vi "Geraete Type ermitteln.vi"(8 "error in (no error)":errorcluster caption="Fehler (Eingang, kein Fehler)", 10 "Istwerte":u16[](array[numeric]), 11 "Steuerung PNS Eingang":refnum<class "Steuerung PNS.lvclass">) -> (0 "error out":errorcluster caption="Fehler (Ausgang)", 2 "Gerätetype":string, 3 "Steuerung PNS Ausgang":refnum<class "Steuerung PNS.lvclass">)   [LabVIEW 2020, in "Steuerung PNS.lvclass"]
uses:
  Steuerung PNS.lvclass
  Steuerung PNS.lvclass/Steuerung PNS.ctl
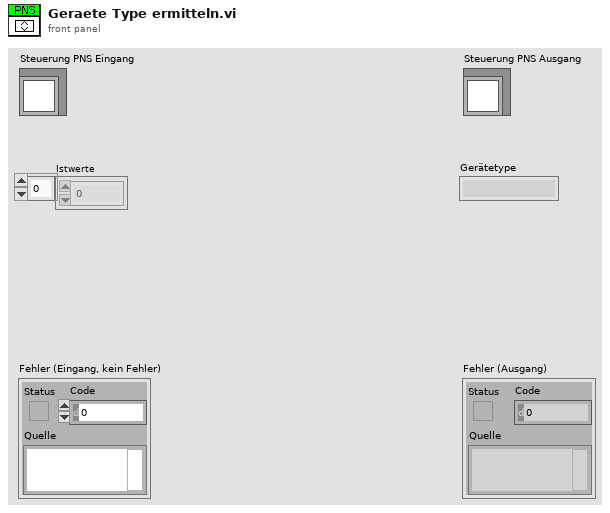
[diagram p1: front panel]
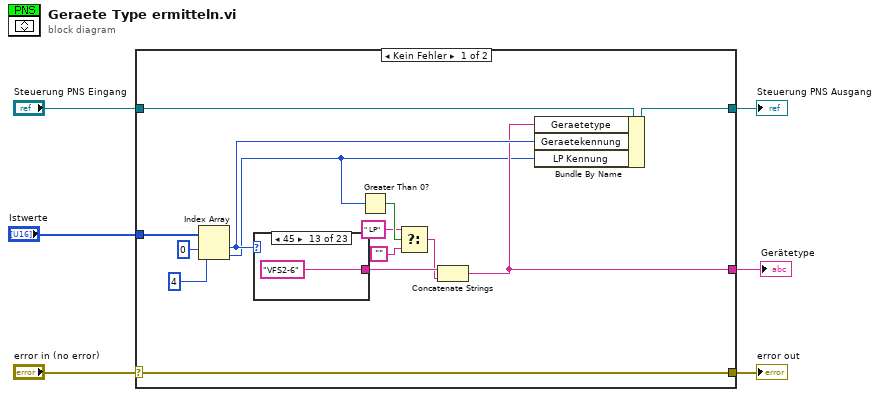
[diagram p0: block diagram]
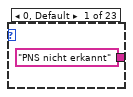
[diagram p2: hidden frame]
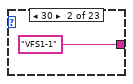
[diagram p3: hidden frame]
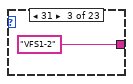
[diagram p4: hidden frame]
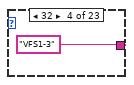
[diagram p5: hidden frame]
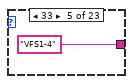
[diagram p6: hidden frame]
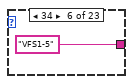
[diagram p7: hidden frame]
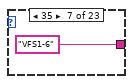
[diagram p8: hidden frame]
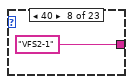
[diagram p9: hidden frame]
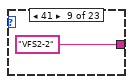
[diagram p10: hidden frame]
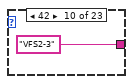
[diagram p11: hidden frame]
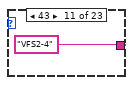
[diagram p12: hidden frame]
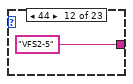
[diagram p13: hidden frame]
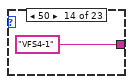
[diagram p14: hidden frame]
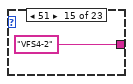
[diagram p15: hidden frame]
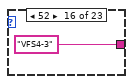
[diagram p16: hidden frame]
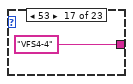
[diagram p17: hidden frame]
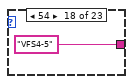
[diagram p18: hidden frame]
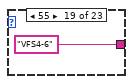
[diagram p19: hidden frame]
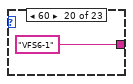
[diagram p20: hidden frame]
diagram:
  n1 = case shown="Kein Fehler" "error in (no error)" {
    selector: "error in (no error)" -> [w19 w46]
    tunnel: [w19 w46] -> w5
    tunnel: [w16 w45] -> w3
    tunnel: "Steuerung PNS Eingang" -> [w20 w45]
    tunnel: "Istwerte" -> [w17 _]
    tunnel: [w12 "PNS nicht erkannt"] -> w1
    frame No Error {
      n2 = Index Array(array=w17, index #1=0 ("Index"), index #2=4 ("Index")) -> (element #1=w14:u16, element #2=w8:u16)
      n3 = case shown="45" w14 {
        tunnel: ["PNS nicht erkannt" "VFS1-1" "VFS1-2" "VFS1-3" "VFS1-4" "VFS1-5" "VFS1-6" "VFS2-1" "VFS2-2" "VFS2-3" "VFS2-4" "VFS2-5" "VFS2-6" "VFS4-1" "VFS4-2" "VFS4-3" "VFS4-4" "VFS4-5" "VFS4-6" "VFS6-1" "VFS6-5" "VFS6-6" "TRE08"] -> w15
        frame 0, Default {
        }
        frame 30 {
        }
        frame 31 {
        }
        frame 32 {
        }
        frame 33 {
        }
        frame 34 {
        }
        frame 35 {
        }
        frame 40 {
        }
        frame 41 {
        }
        frame 42 {
        }
        frame 43 {
        }
        frame 44 {
        }
        frame 45 {
        }
        frame 50 {
        }
        frame 51 {
        }
        frame 52 {
        }
        frame 53 {
        }
        frame 54 {
        }
        frame 55 {
        }
        frame 60 {
        }
        frame 64 {
        }
        frame 65 {
        }
        frame 90 {
        }
      }
      n4 = Greater Than 0?(x=w8) -> (x > 0?=w9:bool)
      n5 = Select(t=" LP", s=w9, f="") -> (s? t:f=w11:string)
      n6 = Concatenate Strings(w15, w11) -> (w12:string)
      n7 = Bundle By Name(cluster=w20, "Geraetetype"=w12, "Geraetekennung"=w14, "LP Kennung"=w8) -> (w16:refnum<class "Steuerung PNS.lvclass">)
    }
    frame Error {
    }
  }
  "error out" <- w5
  "Steuerung PNS Ausgang" <- w3
  "Gerätetype" <- w1
